vi "SRV_Build W,I Command Data.vi"(0 "Motor Control Command":T1={"I2C Address"=0, "Register"=0, "Value"=0, "Active"=TRUE} {"Value" format="%02x"; "Register" format="%02x"; "I2C Address" format="%02x"}) -> (6 "Command Data String":string, 8 "W,I Command Data Field":u8[](array[numeric]) format="%02x", 10 "Active":bool)   [LabVIEW 2014]
doc: "<B>iwabc</B>\nI2C register write ('abc' parameters sent as 8-bit binary)\na is device id, b is register, c is value written to register\n\n\nAuthor: Mike Schultz (LogicPD, Inc)"
uses:
  Motors Config/SRV_Motor Control Command Config.ctl
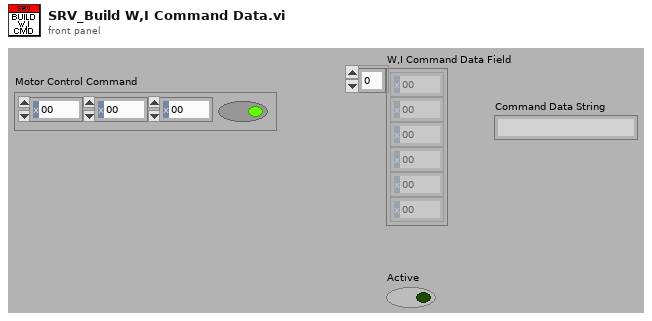
[diagram p1: front panel]
types:
  T1 = typedef "SRV_Motor Control Command Config.ctl" = cluster{"I2C Address":u8, "Register":u8, "Value":u8, "Active":bool}
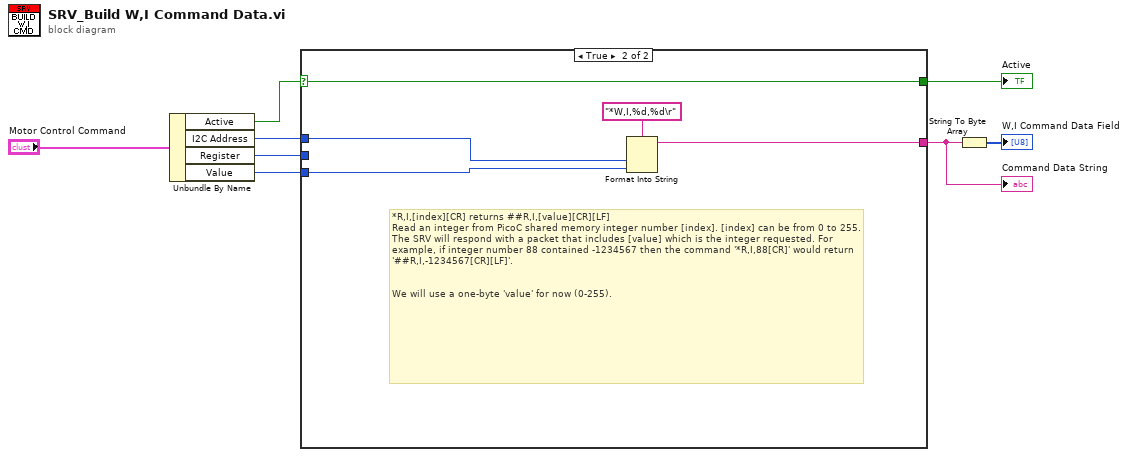
[diagram p0: block diagram]
diagram:
  n1 = Unbundle By Name("Motor Control Command") -> ("Active"=w7:bool, "I2C Address"=w6:u8, "Register"=w5:u8, "Value"=w4:u8)
  n2 = case shown="True" w7 {
    selector: w7 -> [w9 w14]
    tunnel: w6 -> [_ w12]
    tunnel: w5 -> [_ _]
    tunnel: w4 -> [_ w11]
    tunnel: [_ w10] -> w2
    tunnel: [w9 w14] -> w3
    frame False {
    }
    frame True {
      # "*R,I,[index][CR] returns ##R,I,[value][CR][LF]\nRead an integer from PicoC shared memory integer number [index]. [index] can be from 0 to 255. The SRV will respond with a packet that includes [value] which is the integer requested. For example, if integer number 88 contained -1234567 then the command '*R,I,88[CR]' would return '##R,I,-1234567[CR][LF]'.\n\n\nWe will use a one-byte 'value' for now (0-255)."
      n3 = Format Into String(format string="*W,I,%d,%d\r", w12, w11) -> (resulting string=w10:string)  [unwired: 2 in, 1 out]
    }
  }
  "Active" <- w3
  "Command Data String" <- w2
  n4 = String To Byte Array(string=w2) -> (unsigned byte array=→"W,I Command Data Field":u8[])
